vi "ArraySecuence.vi"() -> ()   [LabVIEW 2015]
panel:
  in  "stop":bool
  out "array (last n elements first)":i32[](array[numeric])
  in  "Array":i32[](array[numeric])
  in  "n":i32
  in  "millisecond multiple":u32
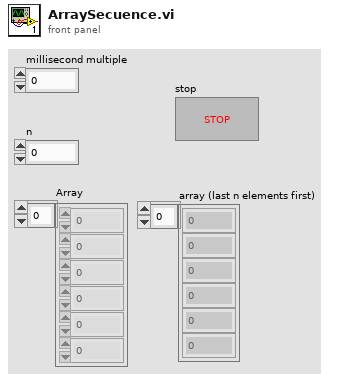
[diagram p1: front panel]
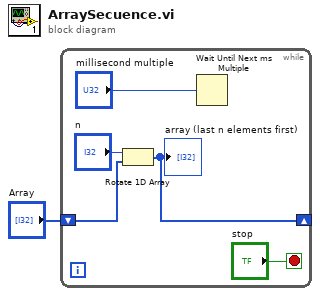
[diagram p0: block diagram]
diagram:
  n1 = while {
    shift-right: [w3] -> _
    shift-left: "Array" -> [w4]
    stop <- "stop" stop-if-true
    n2 = Rotate 1D Array(1:w4, 2:"n") -> (0:w3:i32[])
    "array (last n elements first)" <- w3
    n3 = Wait Until Next ms Multiple(millisecond multiple="millisecond multiple") -> ()  [unwired: 1 out]
  }
